vi "proyecto1 v2.vi"() -> ()   [LabVIEW 2025]
uses:
  <vilib>/MakerHub/LINX/Public/Peripherals/Analog/Analog Read 1 Chan.vi
  <vilib>/MakerHub/LINX/Public/Peripherals/Digital/Digital Read 1 Chan.vi
  <vilib>/MakerHub/LINX/Public/Peripherals/Analog/Analog Read N Chans.vi
  <vilib>/MakerHub/LINX/Public/Peripherals/Digital/Digital Read N Chans.vi
  <vilib>/MakerHub/LINX/Private/Local IO/LinxAnalogRead.vi
  <vilib>/MakerHub/LINX/Public/Utilities/Check Channel.vi
  <vilib>/MakerHub/LINX/Private/Local IO/LinxDigitalRead.vi
  <vilib>/MakerHub/LINX/Public/Utilities/Open Serial.vi
  <vilib>/MakerHub/LINX/Private/Utilties/Generate Error.vi
  <vilib>/express/express shared/transition.llb/Dynamic To Waveform Array.vi
  <vilib>/express/express signal manip/GetorSetDDTAttributes/Set DDT Attributes/SetT0.vi
  <vilib>/express/express shared/transition.llb/Waveform Array To Dynamic.vi
  <vilib>/express/express signal manip/GetorSetDDTAttributes/Set DDT Attributes/Set DDT Properties.xnode
  <vilib>/express/express arith-compare/Formula/XNode/ExpressFormulaBlockNode.xnode
  <vilib>/MakerHub/LINX/LMH-LINX.lvlib
panel:
  out "Oscilograma de Velocidad":dbl(graph)
  out "FL PSI":dbl
  out "FR PSI":dbl
  out "RR PSI":dbl
  out "RL PSI":dbl
  out "Velocidad kilometro/Hora":dbl
  out "Velocidad milla/hora":dbl
  out "RL bar":dbl
  out "RR bar":dbl
  out "FL bar":dbl
  out "FR bar":dbl
  in  "Serial Port":refnum<visa-resource-name>="N/A"
  out "Puerta 3":bool
  out "Puerta 2":bool
  out "Puerta 1":bool
  out "VELOCIDAD":dbl(knob) scale=0.0..240.0
  in  "stop":bool
  out "RL":dbl(knob) scale=0.0..40.0
  out "RR":dbl(knob) scale=0.0..40.0
  out "FL":dbl(knob) scale=0.0..40.0
  out "FR":dbl(knob) scale=0.0..40.0
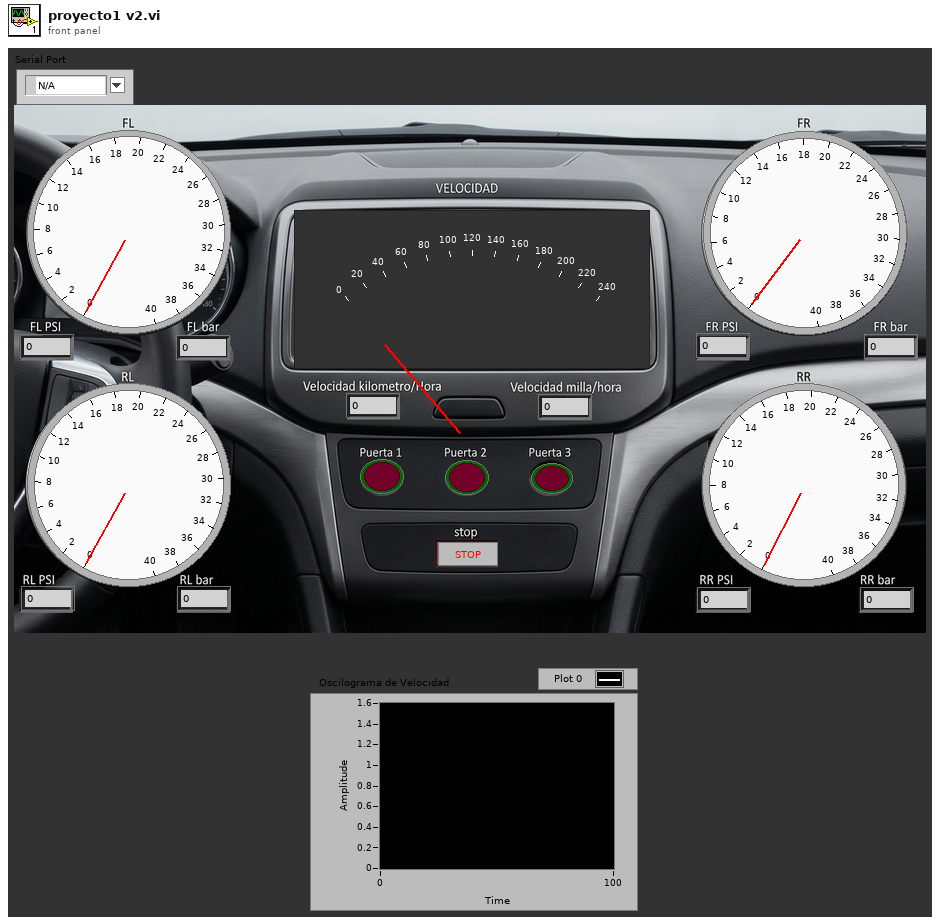
[diagram p1: front panel]
types:
  T1 = typedef "LMH-LINX.lvlib/LINX Ref.ctl" = cluster{"IO":T2, "Interface":T3, "LINX Device Config":T4}
  T2 = typedef "LMH-LINX.lvlib/Platform.ctl" = enum16{"Remote", "Local"}
  T3 = typedef "LMH-LINX.lvlib/Interface.ctl" = enum16{"Serial", "TCP"}
  T4 = typedef "LMH-LINX.lvlib/Device.lvlib/LINX Device Config.ctl" = cluster{"Interface":T3, "COM Port":refnum<visa-resource-name>, "TCP Configuration":T5, "Device Family":u8, "Device ID":u8, "Device Name":string, "TCP Ref":refnum<k5>, "Channels":T6}
  T5 = typedef "LMH-LINX.lvlib/Device.lvlib/TCP Config.ctl" = cluster{"IP Address":string, "Port":u16}
  T6 = typedef "LMH-LINX.lvlib/Channels.ctl" = cluster{"DI":u8[], "DO":u8[], "AI":u8[], "AO":u8[], "PWM":u8[], "QE":u8[], "UART":u8[], "I2C 2":u8[], "SPI":u8[], "CAN":u8[], "Servo":u8[], "AI Ref (V)":dbl, "AI Resolution (Bits)":u8, "AO Ref (V)":dbl, "AO Resolution (Bits)":u8}
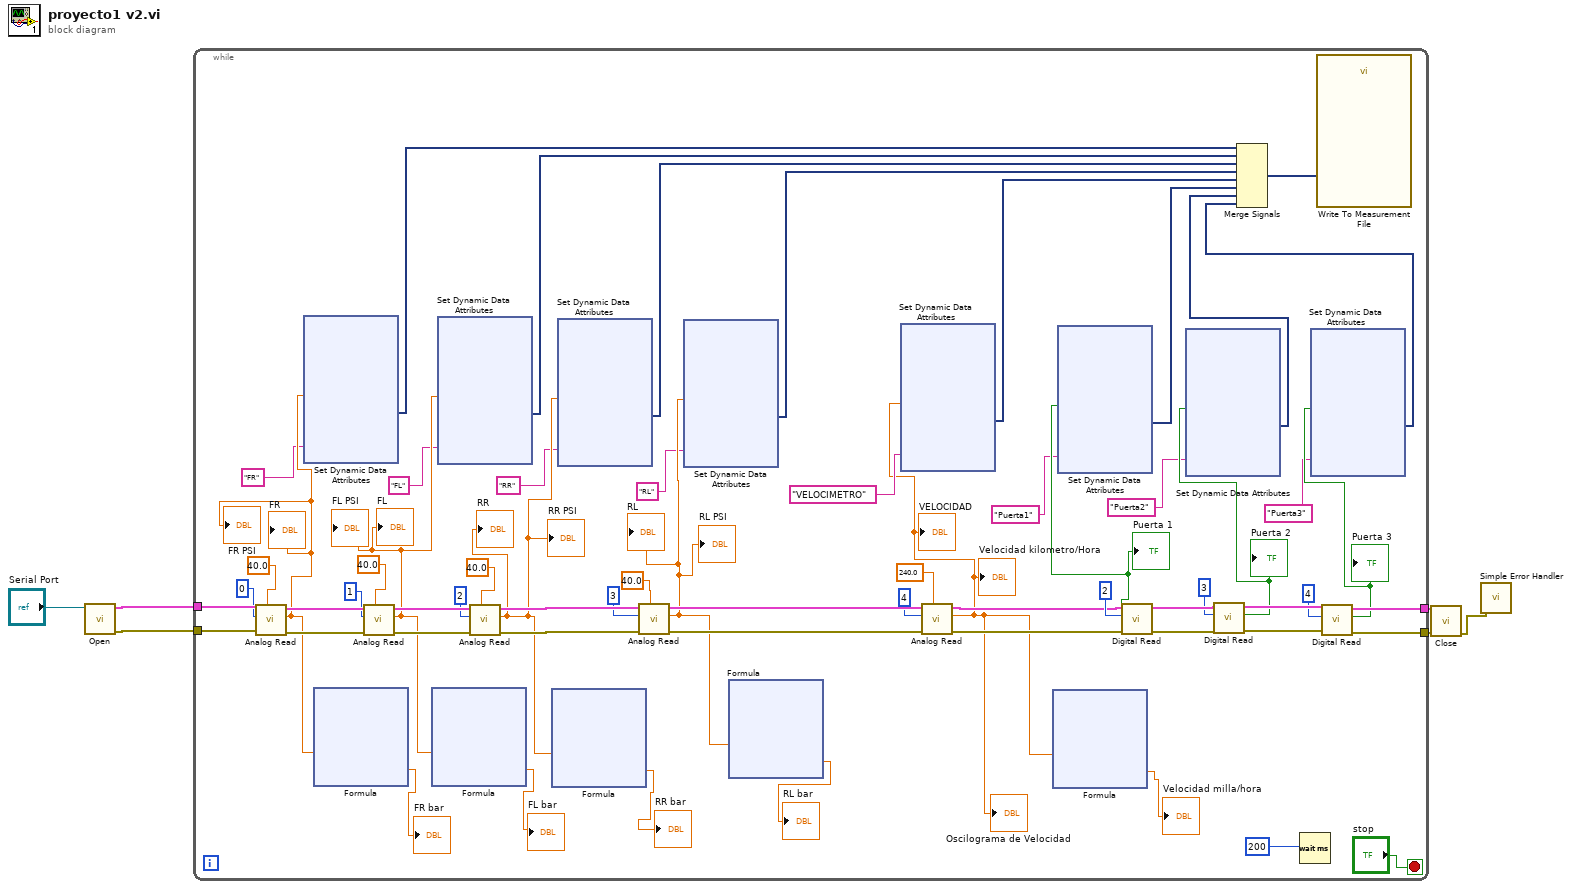
[diagram p0: block diagram]
diagram:
  n1 = call-poly <vilib>:"Open.vi"("Serial Port"="Serial Port") -> ("Error Out"=w3:errorcluster, "LINX Resource"=w4:T1)  [unwired: 8 in, 1 out]
  n2 = while {
    tunnel: w4 -> [w69]
    tunnel: w3 -> [w68]
    tunnel: [w42] -> w2
    tunnel: [w41] -> w1
    stop <- "stop" stop-if-true
    n3 = call-poly <vilib>:"Analog Read.vi"("Analog Ref Override (V)"=40.0, "Error In"=w68, "Analog Channel"=0, "LINX Resource"=w69) -> ("Error Out"=w66:errorcluster, "Voltage"=w30:dbl, "LINX Resource"=w67:T1)  [unwired: 4 in, 1 out]
    "FR" <- w30
    "FR PSI" <- w30
    n4 = xnode "Set Dynamic Data Attributes"("Signals In"=w30, "Signal Name"="FR") -> ("Signals Out"=w29:dynamicdata)  [unwired: 2 in, 1 out]
    n5 = xnode "Formula"("X1"=w30) -> ("Result"=→"FR bar":dbl)  [unwired: 1 in, 1 out]
    n6 = call-poly <vilib>:"Analog Read.vi"("Analog Ref Override (V)"=40.0, "Error In"=w66, "Analog Channel"=1, "LINX Resource"=w67) -> ("Error Out"=w64:errorcluster, "Voltage"=w27:dbl, "LINX Resource"=w65:T1)  [unwired: 4 in, 1 out]
    "FL" <- w27
    "FL PSI" <- w27
    n7 = xnode "Formula"("X1"=w27) -> ("Result"=→"FL bar":dbl)  [unwired: 1 in, 1 out]
    n8 = xnode "Set Dynamic Data Attributes"("Signals In"=w27, "Signal Name"="FL") -> ("Signals Out"=w25:dynamicdata)  [unwired: 2 in, 1 out]
    n9 = call-poly <vilib>:"Analog Read.vi"("Analog Ref Override (V)"=40.0, "Error In"=w64, "Analog Channel"=2, "LINX Resource"=w65) -> ("Error Out"=w62:errorcluster, "Voltage"=w24:dbl, "LINX Resource"=w63:T1)  [unwired: 4 in, 1 out]
    "RR" <- w24
    "RR PSI" <- w24
    n10 = xnode "Formula"("X1"=w24) -> ("Result"=→"RR bar":dbl)  [unwired: 1 in, 1 out]
    n11 = xnode "Set Dynamic Data Attributes"("Signals In"=w24, "Signal Name"="RR") -> ("Signals Out"=w22:dynamicdata)  [unwired: 2 in, 1 out]
    n12 = call-poly <vilib>:"Analog Read.vi"("Analog Ref Override (V)"=40.0, "Error In"=w62, "Analog Channel"=3, "LINX Resource"=w63) -> ("Error Out"=w60:errorcluster, "Voltage"=w21:dbl, "LINX Resource"=w61:T1)  [unwired: 4 in, 1 out]
    "RL" <- w21
    "RL PSI" <- w21
    n13 = xnode "Set Dynamic Data Attributes"("Signals In"=w21, "Signal Name"="RL") -> ("Signals Out"=w19:dynamicdata)  [unwired: 2 in, 1 out]
    n14 = xnode "Formula"("X1"=w21) -> ("Result"=→"RL bar":dbl)  [unwired: 1 in, 1 out]
    n15 = call-poly <vilib>:"Analog Read.vi"("Analog Ref Override (V)"=240.0, "Error In"=w60, "Analog Channel"=4, "LINX Resource"=w61) -> ("Error Out"=w47:errorcluster, "Voltage"=w7:dbl, "LINX Resource"=w31:T1)  [unwired: 4 in, 1 out]
    "VELOCIDAD" <- w7
    "Velocidad kilometro/Hora" <- w7
    "Oscilograma de Velocidad" <- w7
    n16 = xnode "Set Dynamic Data Attributes"("Signals In"=w7, "Signal Name"="VELOCIMETRO") -> ("Signals Out"=w8:dynamicdata)  [unwired: 2 in, 1 out]
    n17 = xnode "Formula"("X1"=w7) -> ("Result"=→"Velocidad milla/hora":dbl)  [unwired: 1 in, 1 out]
    n18 = call-poly <vilib>:"Digital Read.vi"("Error In"=w47, "DI Channel"=2, "LINX Resource"=w31) -> ("Error Out"=w45:errorcluster, "DI Value"=w14:bool, "LINX Resource"=w46:T1)  [unwired: 6 in]
    "Puerta 1" <- w14
    n19 = xnode "Set Dynamic Data Attributes"("Signals In"=w14, "Signal Name"="Puerta1") -> ("Signals Out"=w17:dynamicdata)  [unwired: 2 in, 1 out]
    n20 = call-poly <vilib>:"Digital Read.vi"("Error In"=w45, "DI Channel"=3, "LINX Resource"=w46) -> ("Error Out"=w43:errorcluster, "DI Value"=w13:bool, "LINX Resource"=w44:T1)  [unwired: 6 in]
    "Puerta 2" <- w13
    n21 = xnode "Set Dynamic Data Attributes"("Signals In"=w13, "Signal Name"="Puerta2") -> ("Signals Out"=w16:dynamicdata)  [unwired: 2 in, 1 out]
    n22 = Wait (ms)(milliseconds to wait=u32 200 ("millisecond timer value")) -> ()  [unwired: 1 out]
    n23 = call-poly <vilib>:"Digital Read.vi"("Error In"=w43, "DI Channel"=4, "LINX Resource"=w44) -> ("Error Out"=w42:errorcluster, "DI Value"=w12:bool, "LINX Resource"=w41:T1)  [unwired: 6 in]
    "Puerta 3" <- w12
    n24 = xnode "Set Dynamic Data Attributes"("Signals In"=w12, "Signal Name"="Puerta3") -> ("Signals Out"=w15:dynamicdata)  [unwired: 2 in, 1 out]
    n25 = Merge Signals(w29, w25, w22, w19, w8, w17, w16, w15) -> (w37:dynamicdata)
    n26 = call "Write To Measurement File"("Signals"=w37) -> ()  [unwired: 16 in, 3 out]
  }
  n27 = call <vilib>:"Close.vi"("Error In"=w2, "LINX Resource"=w1) -> ("Error Out"=w5:errorcluster)  [unwired: 9 in]
  n28 = call <vilib>:"Simple Error Handler.vi"("error in (no error)"=w5) -> ()  [unwired: 4 in, 5 out]
